vi "sub vi - cycle&temp fail v4.vi"(0 "Amps Lo?":bool, 2 "Input Cluster":T1, 3 "SELECT":T2(ring), 4 "Amps Hi?":bool, 5 "Result In":bool) -> (15 "(FAIL) out":cluster{"FAIL LO":dbl, "FAIL HI":dbl}, 16 "(DISP) out":T3, 18 "Result Out":bool, 19 "file error":errorcluster)   [LabVIEW 2013]
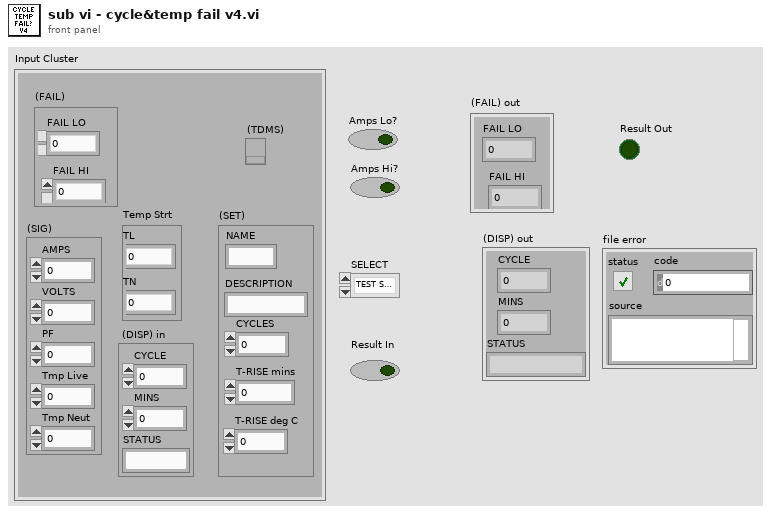
[diagram p1: front panel]
types:
  T1 = cluster{"(FAIL)":cluster{"FAIL LO":dbl, "FAIL HI":dbl}, "(SIG)":cluster{"AMPS":dbl, "VOLTS":dbl, "PF":dbl, "Tmp Live":dbl, "Tmp Neut":dbl}, "Temp Strt":cluster{"TL":dbl, "TN":dbl}, " (DISP) in":cluster{"CYCLE":dbl, "MINS":dbl, "STATUS":string}, "(SET)":cluster{"NAME":string, "DESCRIPTION":string, "CYCLES":dbl, "T-RISE mins":dbl, "T-RISE deg C":dbl}, "(TDMS)":refnum<k34>}
  T2 = enum32{"TEST SET UP", "CYCLE TEST", "T-RISE TEST"}
  T3 = cluster{"CYCLE":dbl, "MINS":dbl, "STATUS":string}
  T4 = cluster{"AMPS":dbl, "VOLTS":dbl, "PF":dbl, "Tmp Live":dbl, "Tmp Neut":dbl}
  T5 = cluster{"NAME":string, "DESCRIPTION":string, "CYCLES":dbl, "T-RISE mins":dbl, "T-RISE deg C":dbl}
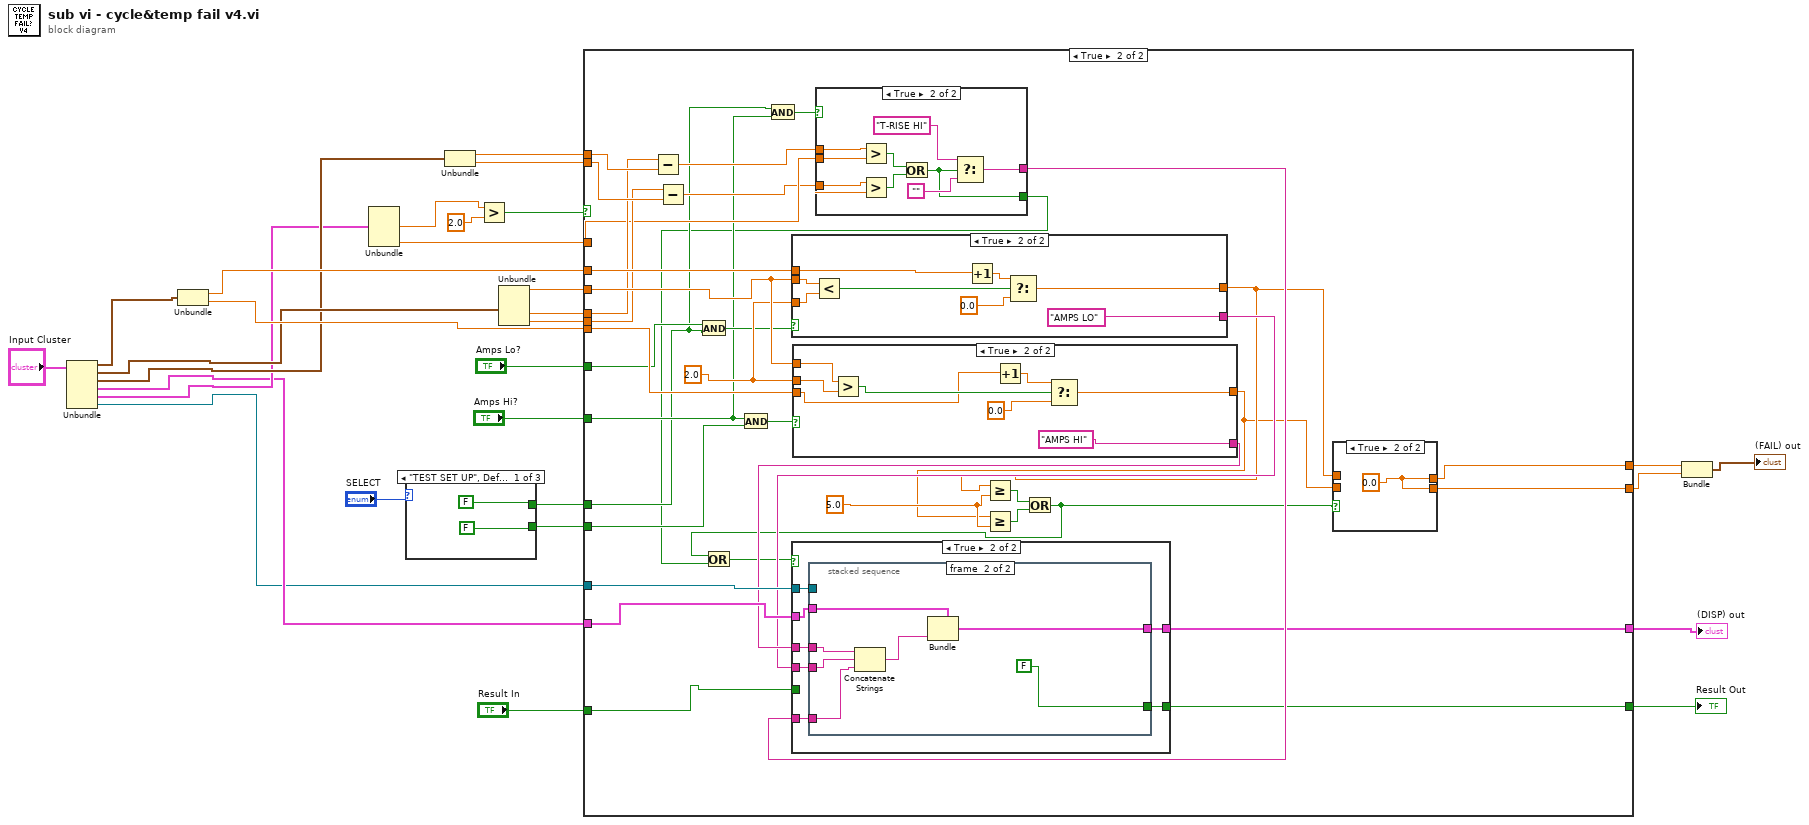
[diagram p0: block diagram]
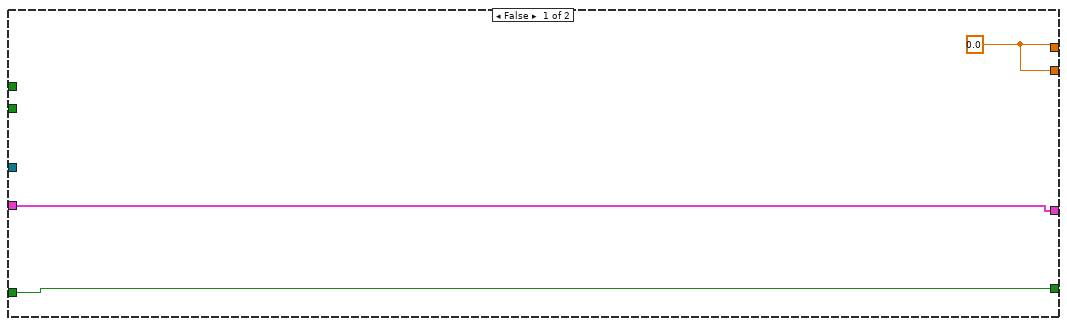
[diagram p2: hidden frame]
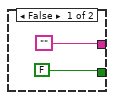
[diagram p4: hidden frame]
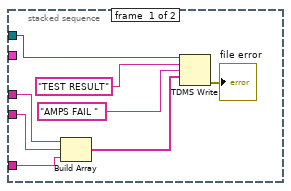
[diagram p6: hidden frame]
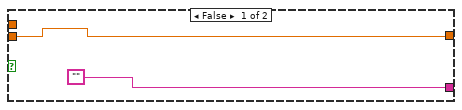
[diagram p7: hidden frame]
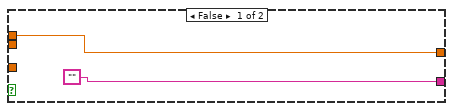
[diagram p8: hidden frame]
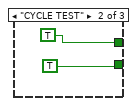
[diagram p9: hidden frame]
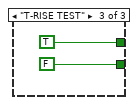
[diagram p10: hidden frame]
diagram:
  n1 = Unbundle("Input Cluster") -> ("(FAIL)"=w14:cluster{"FAIL LO":dbl, "FAIL HI":dbl}, "(SIG)"=w11:T4, "Temp Strt"=w10:cluster{"TL":dbl, "TN":dbl}, "(DISP) in"=w8:T3, "(SET)"=w9:T5, "(TDMS)"=w7:refnum<k34>)
  n2 = Unbundle(w14) -> ("FAIL LO"=w13:dbl, "FAIL HI"=w12:dbl)
  n3 = Unbundle(w9) -> ("CYCLES"=w18:dbl, "T-RISE deg C"=w23:dbl)  [unwired: 3 out]
  n4 = case shown="\"TEST SET UP\", Default" "SELECT" {
    tunnel: [FALSE TRUE TRUE] -> w19
    tunnel: [FALSE TRUE FALSE] -> w22
    frame "TEST SET UP", Default {
    }
    frame "CYCLE TEST" {
    }
    frame "T-RISE TEST" {
    }
  }
  n5 = Unbundle(w10) -> ("TL"=w27:dbl, "TN"=w26:dbl)
  n6 = Greater?(x=w18, y=2.0) -> (0:w16:bool)
  n7 = Unbundle(w11) -> ("AMPS"=w28:dbl, "Tmp Live"=w25:dbl, "Tmp Neut"=w24:dbl)  [unwired: 2 out]
  n8 = case shown="True" w16 {
    tunnel: w28 -> [_ w74]
    tunnel: w13 -> [_ w72]
    tunnel: w12 -> [_ w71]
    tunnel: w7 -> [_ w70]
    tunnel: w8 -> [w37 w69]
    tunnel: w27 -> [_ w68]
    tunnel: w26 -> [_ w67]
    tunnel: w25 -> [_ w66]
    tunnel: w24 -> [_ w65]
    tunnel: w23 -> [_ w64]
    tunnel: w22 -> [_ w54]
    tunnel: "Amps Lo?" -> [_ w52]
    tunnel: "Amps Hi?" -> [_ w50]
    tunnel: w19 -> [_ w49]
    tunnel: [w38 w46] -> w5
    tunnel: [w38 w45] -> w4
    tunnel: [w37 w44] -> w3
    tunnel: [w36 w43] -> w2
    tunnel: "Result In" -> [w36 w42]
    frame False {
      w38 = 0.0
    }
    frame True {
      w57 = 5.0
      w73 = 2.0
      n9 = Subtract(x=w66, y=w68) -> (x-y=w63:dbl)
      n10 = Subtract(x=w65, y=w67) -> (x-y=w62:dbl)
      n11 = And(x=w52, y=w49) -> (x .and. y?=w53:bool)
      n12 = And(x=w50, y=w54) -> (x .and. y?=w55:bool)
      n13 = And(x=w49, y=w50) -> (x .and. y?=w51:bool)
      n14 = case shown="True" w53 {
        tunnel: w74 -> [_ w132]
        tunnel: ["" "AMPS LO"] -> w60
        tunnel: w73 -> [_ w130]
        tunnel: w72 -> [w123 w126]
        tunnel: [w123 w125] -> w48
        frame False {
        }
        frame True {
          n15 = Less?(x=w132, y=w130) -> (x < y?=w129:bool)
          n16 = Increment(x=w126) -> (x+1=w128:dbl)
          n17 = Select(t=w128, s=w129, f=0.0) -> (s? t:f=w125:dbl)
        }
      }
      n18 = case shown="True" w55 {
        tunnel: w74 -> [_ w122]
        tunnel: ["" "AMPS HI"] -> w61
        tunnel: w73 -> [_ w120]
        tunnel: [w113 w116] -> w47
        tunnel: w71 -> [w113 w115]
        frame False {
        }
        frame True {
          n19 = Greater?(x=w122, y=w120) -> (0:w119:bool)
          n20 = Increment(x=w115) -> (x+1=w118:dbl)
          n21 = Select(t=w118, s=w119, f=0.0) -> (s? t:f=w116:dbl)
        }
      }
      n22 = case shown="True" w51 {
        tunnel: w64 -> [_ w88]
        tunnel: w63 -> [_ w87]
        tunnel: w62 -> [_ w86]
        tunnel: ["" w81] -> w56
        tunnel: [FALSE w80] -> w40
        frame False {
        }
        frame True {
          n23 = Greater?(x=w87, y=w88) -> (0:w84:bool)
          n24 = Greater?(x=w86, y=w88) -> (0:w85:bool)
          n25 = Or(x=w84, y=w85) -> (x .or. y?=w80:bool)
          n26 = Select(t="T-RISE HI", s=w80, f="") -> (s? t:f=w81:string)
        }
      }
      n27 = Greater Or Equal?(x=w48, y=w57) -> (x >= y?=w59:bool)
      n28 = Greater Or Equal?(x=w47, y=w57) -> (x >= y?=w58:bool)
      n29 = Or(x=w59, y=w58) -> (x .or. y?=w41:bool)
      n30 = Or(x=w41, y=w40) -> (x .or. y?=w39:bool)
      n31 = case shown="True" w39 {
        tunnel: w61 -> [_ w97]
        tunnel: w60 -> [_ w96]
        tunnel: w69 -> [w90 w95]
        tunnel: w70 -> [_ w94]
        tunnel: w56 -> [_ w93]
        tunnel: [w90 w92] -> w44
        tunnel: [w89 w91] -> w43
        tunnel: w42 -> [w89 _]
        frame False {
        }
        frame True {
          n32 = stacked-sequence {
            tunnel: w97 -> [w104 w112]
            tunnel: w96 -> [w103 w111]
            tunnel: w95 -> [_ w109]
            tunnel: w94 -> [w99 _]
            tunnel: w93 -> [w98 w108]
            tunnel: [_ w107] -> w92
            tunnel: [_ FALSE] -> w91
            frame #0 {
              n33 = Build Array(w104, w103, w98) -> (w102:string[])
              n34 = TDMS Write(0:w99, 5:"TEST RESULT", 7:"AMPS FAIL ", 9:w102) -> (15:→"file error":errorcluster)  [unwired: 2 in, 3 out]
            }
            frame #1 {
              n35 = Concatenate Strings(w112, w111, w108) -> (w110:string)
              n36 = Bundle(cluster=w109, "STATUS"=w110) -> (w107:T3)  [unwired: 2 in]
            }
          }
        }
      }
      n37 = case shown="True" w41 {
        tunnel: w48 -> [w76 _]
        tunnel: w47 -> [w75 _]
        tunnel: [w76 w77] -> w46
        tunnel: [w75 w77] -> w45
        frame False {
        }
        frame True {
          w77 = 0.0
        }
      }
    }
  }
  "(DISP) out" <- w3
  "Result Out" <- w2
  n38 = Bundle("FAIL LO"=w5, "FAIL HI"=w4) -> (→"(FAIL) out":cluster{"FAIL LO":dbl, "FAIL HI":dbl})  [unwired: 1 in]
